vi "DP-Restore Defaults.vi"() -> (8 "Parameters":T1={"Stimulus"={"Ear"=enum."Right", "f2 freqs (kHz)"="", "Start (dB)"=16.0, "Stop (dB)"=30.0, "Step (dB)"=0.0, "Mode"=enum."L1 = L2", "override recal"=FALSE, "Sampling Rate (Hz)"=5.0, "Frame (ms)"=0.0}, "Response"={"Time avgs"=25000, "Freq avgs"=100000, "Mic gain (dB)"=5.0, "Save raw"=FALSE}}, 15 "error out":errorcluster)   [LabVIEW 2020]
uses:
  Typedefs/DP-Parameters.ctl
  Typedefs/DP-Stimulus Params.ctl
  Typedefs/DP-Response Params.ctl
panel:
  in  "Defaults":T1={"Stimulus"={"Ear"=enum."Right", "f2 freqs (kHz)"="5.6;8.0;11.3;16;22.6;32;", "Start (dB)"=20.0, "Stop (dB)"=80.0, "Step (dB)"=5.0, "Mode"=enum."L1 = L2 + 10 dB", "override recal"=FALSE, "Sampling Rate (Hz)"=200000.0, "Frame (ms)"=50.0}, "Response"={"Time avgs"=8, "Freq avgs"=4, "Mic gain (dB)"=40.0, "Save raw"=FALSE}}
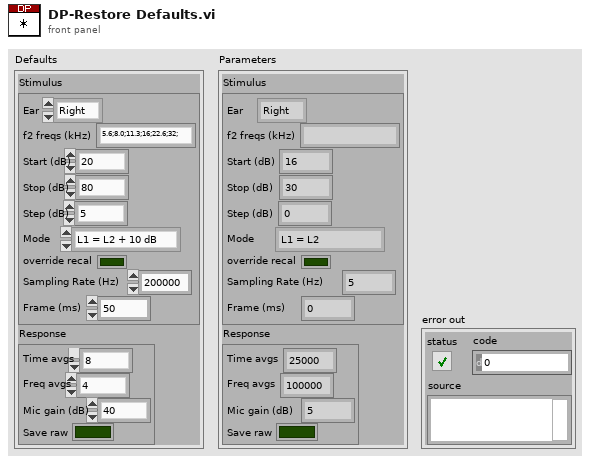
[diagram p1: front panel]
types:
  T1 = typedef "DP-Parameters.ctl" = cluster{"Stimulus":T2, "Response":T3}
  T2 = typedef "DP-Stimulus Params.ctl" = cluster{"Ear":enum16{"Right", "Left"}, "f2 freqs (kHz)":string, "Start (dB)":dbl, "Stop (dB)":dbl, "Step (dB)":dbl, "Mode":enum16{"L1 = L2", "L1 = L2 + 10 dB"}, "override recal":bool, "Sampling Rate (Hz)":dbl, "Frame (ms)":dbl}
  T3 = typedef "DP-Response Params.ctl" = cluster{"Time avgs":i32, "Freq avgs":i32, "Mic gain (dB)":dbl, "Save raw":bool}
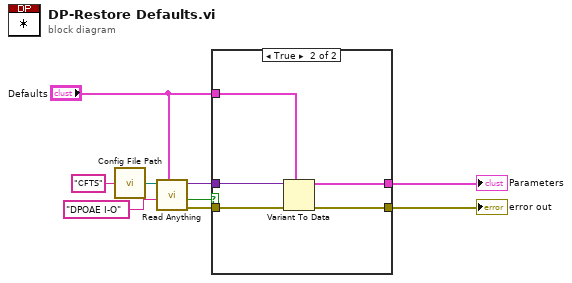
[diagram p0: block diagram]
diagram:
  n1 = call "Config File Path.vi"("AppName"="CFTS") -> ("Default config file name"=w3:path)
  n2 = call "Read Anything.vi"("Type of Anything"="Defaults", "Section Name (Name of \"Type of Anything\")"="DPOAE I-O" ("Section Name (Name of \"Type of Anything\")"), "Path (dialog)"=w3) -> ("Error Out"=w7:errorcluster, "Found?"=w6:bool, "Anything"=w9:variant)  [unwired: 6 in]
  n3 = case shown="True" w6 {
    tunnel: w9 -> [_ w16]
    tunnel: "Defaults" -> [w10 w15]
    tunnel: w7 -> [w11 w14]
    tunnel: [w10 w13] -> w2
    tunnel: [w11 w12] -> w1
    frame False {
    }
    frame True {
      n4 = Variant To Data(error in=w14, type=w15, Variant=w16) -> (data=w13:T1, error out=w12:errorcluster)
    }
  }
  "Parameters" <- w2
  "error out" <- w1
